vi "AlliGator Get IRF Values & Locations.vi"(10 "[IRF Data]":dbl[][](array[numeric])) -> (0 "IRF Locations":cluster{"X":i32, "Y":i32}[](array[cluster]), 1 "[IRF Values]":dbl[][](array[numeric]))   [LabVIEW 2021, in "AlliGator Decay Analysis.lvlib" / "AlliGator Decay Fit.lvlib"]
doc: "Gets the array of stored <B>IRF Values</B> as well as the <B>IRF Locations</B>."
uses:
  AlliGator Decay Fit.lvlib
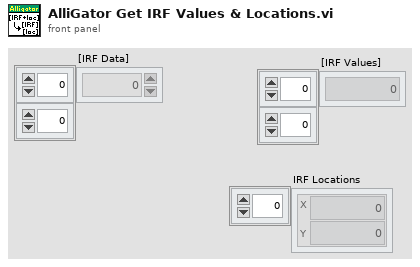
[diagram p1: front panel]
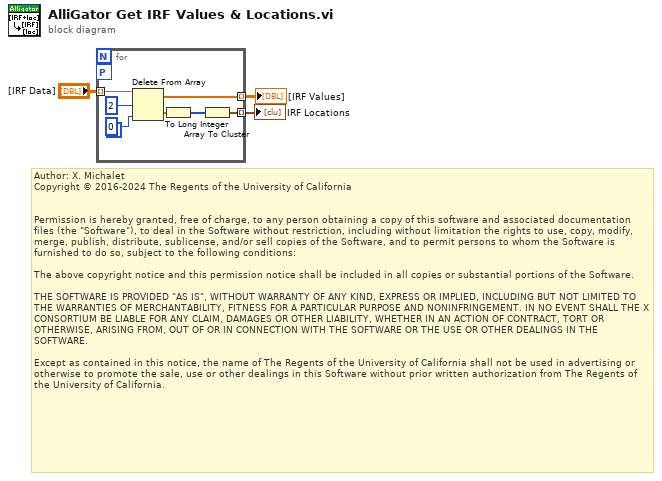
[diagram p0: block diagram]
diagram:
  # "Author: X. Michalet\nCopyright © 2016-2024 The Regents of the University of California\n \n\nPermission is hereby granted, free of charge, to any person obtaining a copy of this software and associated documentation files (the \"Software\"), to deal in the Software without restriction, including without limitation the rights to use, copy, modify, merge, publish, distribute, sublicense, and/or sell copies of the Software, and to permit persons to whom the Software is furnished to do so, subject to the following conditions:\n\nThe above copyright notice and this permission notice shall be included in all copies or substantial portions of the Software.\n\nTHE SOFTWARE IS PROVIDED \"AS IS\", WITHOUT WARRANTY OF ANY KIND, EXPRESS OR IMPLIED, INCLUDING BUT NOT LIMITED TO THE WARRANTIES OF MERCHANTABILITY, FITNESS FOR A PARTICULAR PURPOSE AND NONINFRINGEMENT. IN NO EVENT SHALL THE X CONSORTIUM BE LIABLE FOR ANY CLAIM, DAMAGES OR OTHER LIABILITY, WHETHER IN AN ACTION OF CONTRACT, TORT OR OTHERWISE, ARISING FROM, OUT OF OR IN CONNECTION WITH THE SOFTWARE OR THE USE OR OTHER DEALINGS IN THE SOFTWARE.\n\nExcept as contained in this notice, the name of The Regents of the University of California shall not be used in advertising or otherwise to promote the sale, use or other dealings in this Software without prior written authorization from The Regents of the University of California."
  n1 = for {
    tunnel: "[IRF Data]" -> [w8] mode=indexing
    tunnel: [w7] -> w2 mode=indexing
    tunnel: [w5] -> w1 mode=indexing
    workers-P: _ -> [_]
    n2 = Delete From Array(array=w8, length=2, index=0) -> (deleted portion=w6:dbl[], array with subset deleted=w7:dbl[])
    n3 = To Long Integer(number=w6) -> (32bit integer=w4:i32[])
    n4 = Array To Cluster(array=w4) -> (cluster=w5:cluster{"[0]":i32, "[1]":i32})
  }
  "[IRF Values]" <- w2
  "IRF Locations" <- w1
